vi "readAimingBeamSetting.vi"(8 "error in (no error)":errorcluster) -> (0 "error out":errorcluster, 3 "Aiming Beam Setting":T1={"Aiming Beam COM Port"="COM3", "Min Current"=0.0, "Max Current"=63.0, "Default Current"=20.0, "Frequency(Hz)"=15})   [LabVIEW 2020]
uses:
  SubVI/TecLaserControl/AimingBeam.ctl
  <vilib>/Utility/config.llb/Read Key (String).vi
  <vilib>/Utility/config.llb/Read Key (Double).vi
  <vilib>/Utility/config.llb/Read Key (I32).vi
  <vilib>/Utility/config.llb/NI_LVConfig.lvlib
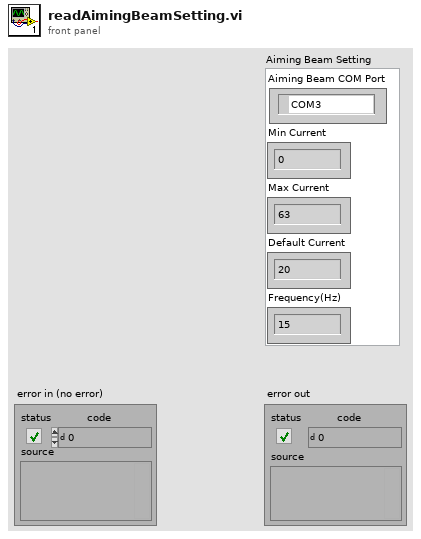
[diagram p1: front panel]
types:
  T1 = typedef "AimingBeam.ctl" = cluster{"Aiming Beam COM Port":refnum<visa-resource-name>, "Min Current":dbl, "Max Current":dbl, "Default Current":dbl, "Frequency(Hz)":u32}
  T2 = typedef "NI_LVConfig.lvlib/Config Data RefNum.ctl" = refnum<k1>
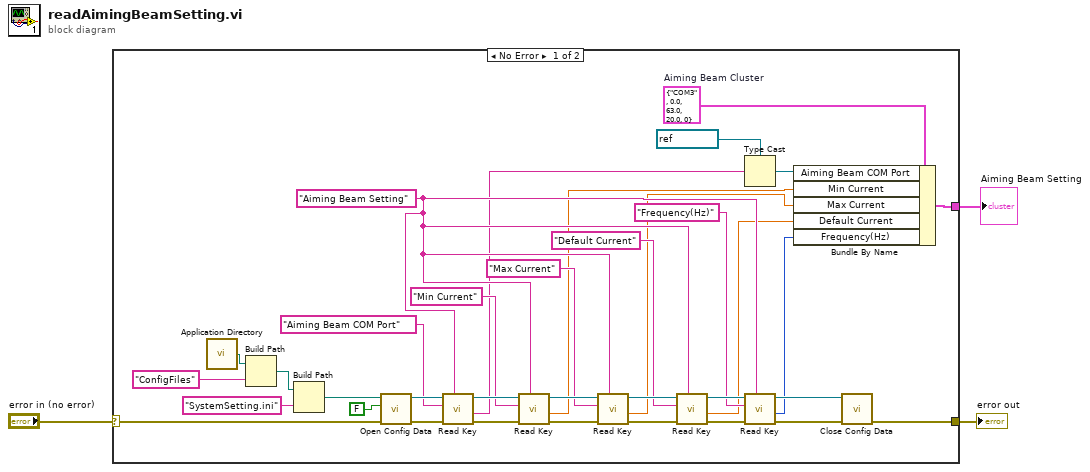
[diagram p0: block diagram]
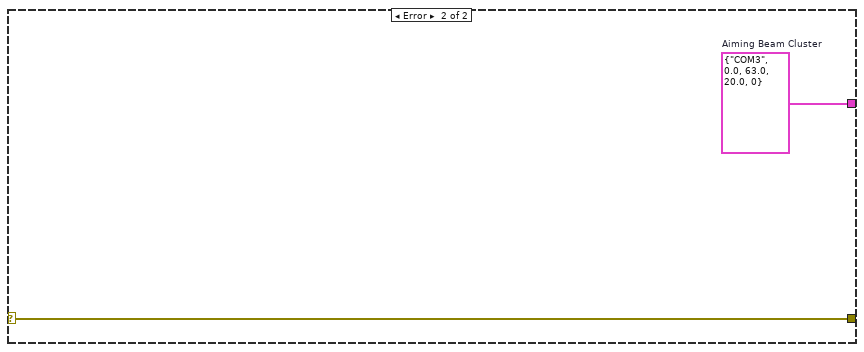
[diagram p2: hidden frame]
diagram:
  n1 = case shown="No Error" "error in (no error)" {
    selector: "error in (no error)" -> [w32 w40]
    tunnel: [w18 w40] -> w2
    tunnel: [w7 w39] -> w1
    frame No Error {
      w17 = "Aiming Beam Setting" ("section")
      w12 = T1 {"Aiming Beam COM Port"="COM3", "Min Current"=0.0, "Max Current"=63.0, "Default Current"=20.0, "Frequency(Hz)"=0}  # Aiming Beam Cluster
      n2 = call <vilib>:"Application Directory.vi"() -> ("Application Directory"=w38:path)
      n3 = Build Path(base path=w38, name or relative path="ConfigFiles") -> (appended path=w36:path)
      n4 = Build Path(base path=w36, name or relative path="SystemSetting.ini") -> (appended path=w34:path)
      n5 = call <vilib>:"Open Config Data.vi"("error in (no error)"=w32, "create file if necessary (T)"=FALSE, "configuration file path"=w34) -> ("error out"=w30:errorcluster, "refnum"=w31:T2)  [unwired: 6 in, 1 out]
      n6 = call-poly <vilib>:"Read Key.vi"("section"=w17, "error in (no error)"=w30, "key"="Aiming Beam COM Port", "refnum"=w31) -> ("error out"=w24:errorcluster, "value"=w6:string, "refnum out"=w28:T2)  [unwired: 4 in, 1 out]
      n7 = call-poly <vilib>:"Read Key.vi"("section"=w17, "error in (no error)"=w24, "key"="Min Current", "refnum"=w28) -> ("error out"=w23:errorcluster, "value"=w11:dbl, "refnum out"=w27:T2)  [unwired: 4 in, 1 out]
      n8 = call-poly <vilib>:"Read Key.vi"("section"=w17, "error in (no error)"=w23, "key"="Max Current", "refnum"=w27) -> ("error out"=w22:errorcluster, "value"=w10:dbl, "refnum out"=w26:T2)  [unwired: 4 in, 1 out]
      n9 = call-poly <vilib>:"Read Key.vi"("section"=w17, "error in (no error)"=w22, "key"="Default Current", "refnum"=w26) -> ("error out"=w21:errorcluster, "value"=w9:dbl, "refnum out"=w25:T2)  [unwired: 4 in, 1 out]
      n10 = Type Cast(type=refnum<visa-resource-name> "COM3" ("Aiming Beam COM Port"), x=w6) -> (*(type *) &x=w4:refnum<visa-resource-name>)
      n11 = call-poly <vilib>:"Read Key.vi"("section"=w17, "error in (no error)"=w21, "key"="Frequency(Hz)", "refnum"=w25) -> ("error out"=w19:errorcluster, "value"=w8:i32, "refnum out"=w20:T2)  [unwired: 4 in, 1 out]
      n12 = Bundle By Name(cluster=w12, "Aiming Beam COM Port"=w4, "Min Current"=w11, "Max Current"=w10, "Default Current"=w9, "Frequency(Hz)"=w8) -> (w7:T1)
      n13 = call <vilib>:"Close Config Data.vi"("error in (no error)"=w19, "refnum"=w20) -> ("error out"=w18:errorcluster)  [unwired: 8 in, 1 out]
    }
    frame Error {
      w39 = T1 {"Aiming Beam COM Port"="COM3", "Min Current"=0.0, "Max Current"=63.0, "Default Current"=20.0, "Frequency(Hz)"=0}  # Aiming Beam Cluster
    }
  }
  "error out" <- w2
  "Aiming Beam Setting" <- w1
